vi "Client LabVIEW.vi"() -> ()   [LabVIEW 2014]
panel:
  out "ERROR":string
  out "Comptador":dbl
  out "Mínim":dbl
  out "Mitjana":dbl
  out "Waveform Chart":T1(graph)
  out "Màxim":dbl
  in  "Enviar missatge":bool
  in  "Marxa/parada":bool
  in  "Nº mostres":i32
  in  "Temps":i32 format="%02d"
  in  "Escull una acció":T2(ring)
  out "Missatge del servidor":string
  # "Marxa"
  # "Parada"
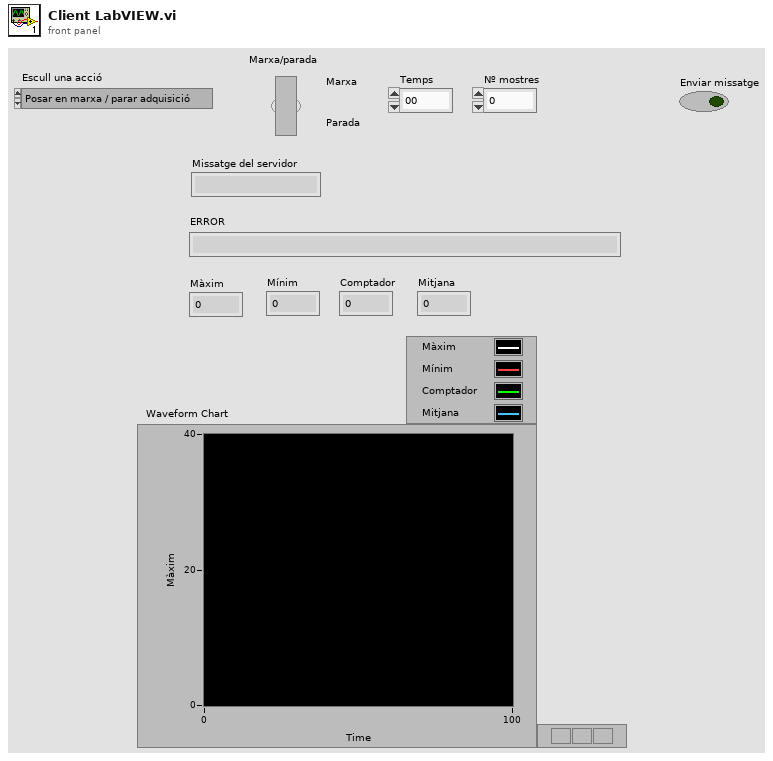
[diagram p1: front panel]
types:
  T1 = cluster{"Màxim":dbl, "Mínim":dbl, "Comptador":dbl, "Mitjana":dbl}
  T2 = enum16{"Posar en marxa / parar adquisició", "Demanar la mitjana", "Demanar màxim", "Demanar mínim", "Reset màxim/mínim", " Nombre de mostres guardades"}
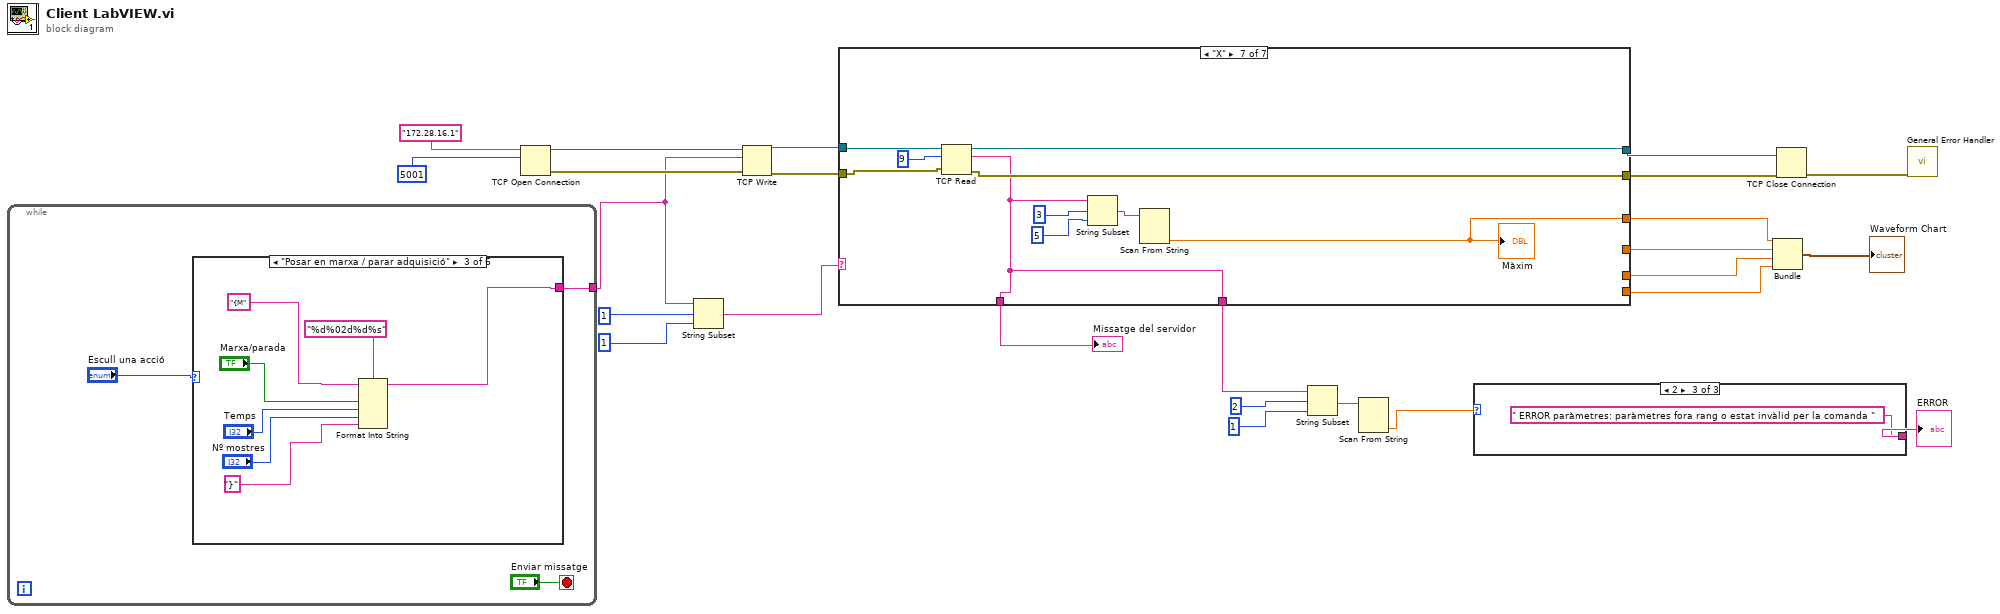
[diagram p0: block diagram]
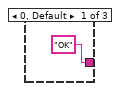
[diagram p2: hidden frame]
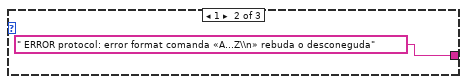
[diagram p3: hidden frame]
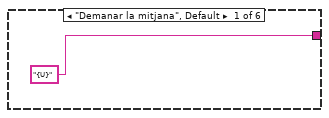
[diagram p4: hidden frame]
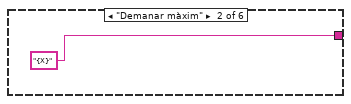
[diagram p5: hidden frame]
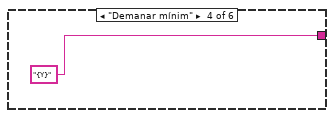
[diagram p6: hidden frame]
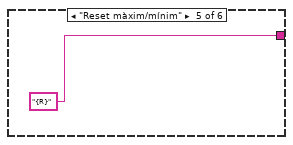
[diagram p7: hidden frame]
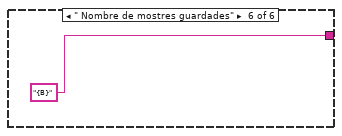
[diagram p8: hidden frame]
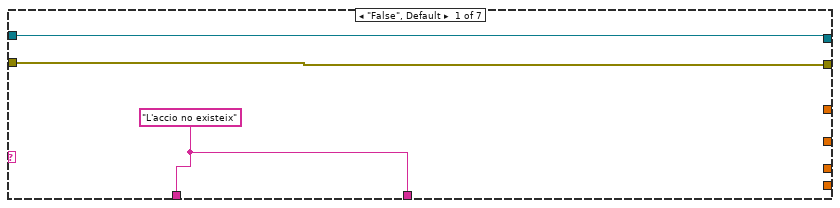
[diagram p9: hidden frame]
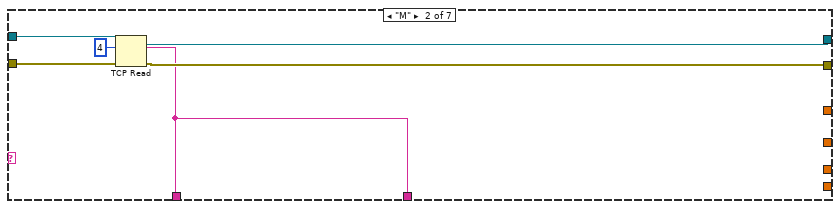
[diagram p10: hidden frame]
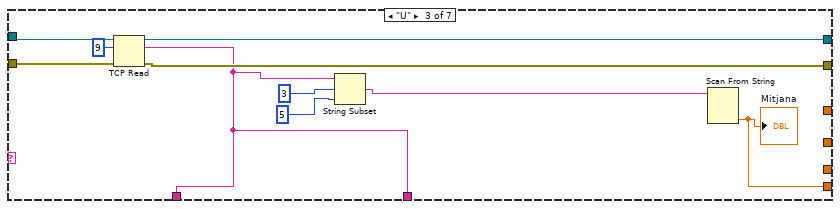
[diagram p11: hidden frame]
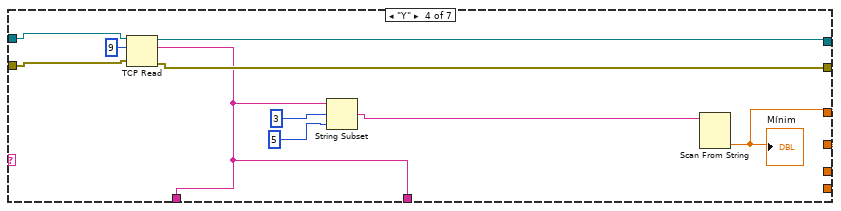
[diagram p12: hidden frame]
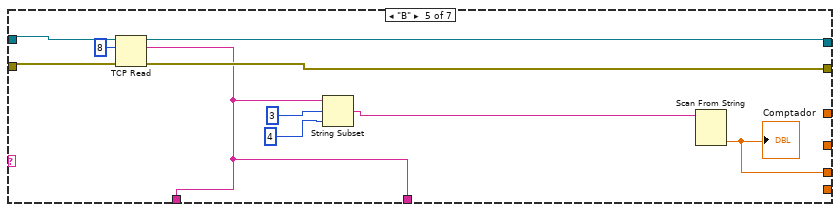
[diagram p13: hidden frame]
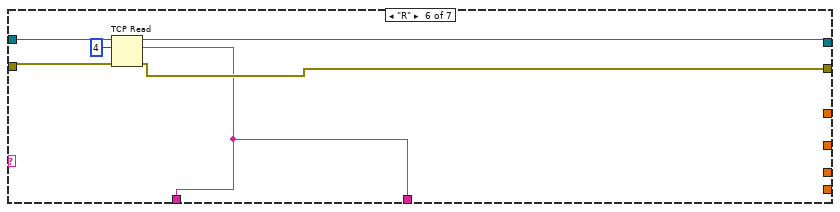
[diagram p14: hidden frame]
diagram:
  n1 = while {
    tunnel: [w27] -> w13
    stop <- "Enviar missatge" stop-if-true
    n2 = case shown="\"Posar en marxa / parar adquisició\"" "Escull una acció" {
      tunnel: ["{U}" "{X}" w31 "{Y}" "{R}" "{B}"] -> w27
      frame "Demanar la mitjana", Default {
      }
      frame "Demanar màxim" {
      }
      frame "Posar en marxa / parar adquisició" {
        n3 = Format Into String(format string="%d%02d%d%s", initial string="{M", "Marxa/parada", "Temps", "Nº mostres", "}") -> (resulting string=w31:string)  [unwired: 1 in, 1 out]
      }
      frame "Demanar mínim" {
      }
      frame "Reset màxim/mínim" {
      }
      frame " Nombre de mostres guardades" {
      }
    }
  }
  n4 = TCP Open Connection(address="172.28.16.1", remote port or service name=u16 5001) -> (connection ID=w23:refnum<k5>, error out=w22:errorcluster)  [unwired: 3 in]
  n5 = String Subset(string=w13, offset (0)=1, length (rest)=1 ("length (rest)")) -> (substring=w19:string)
  n6 = TCP Write(connection ID=w23, data in=w13, error in (no error)=w22) -> (connection ID out=w18:refnum<k5>, error out=w17:errorcluster)  [unwired: 1 in, 1 out]
  n7 = case shown="\"X\"" w19 {
    tunnel: w18 -> [w43 w48 w58 w68 w78 w84 w94]
    tunnel: w17 -> [w42 w47 w57 w67 w77 w83 w93]
    tunnel: [w43 w46 w55 w66 w76 w82 w92] -> w16
    tunnel: [w42 w45 w56 w65 w75 w81 w91] -> w15
    tunnel: [w41 w44 w51 w61 w71 w80 w87] -> w12
    tunnel: [w41 w44 w51 w61 w71 w80 w87] -> w8
    tunnel: [_ _ _ _ _ _ w86] -> w5
    tunnel: [_ _ _ w60 _ _ _] -> w4
    tunnel: [_ _ _ _ w70 _ _] -> w3
    tunnel: [_ _ w50 _ _ _ _] -> w2
    frame "False", Default {
      w41 = "L'accio no existeix" ("data out")
    }
    frame "M" {
      n8 = TCP Read(connection ID=w48, bytes to read=4, error in (no error)=w47) -> (connection ID out=w46:refnum<k5>, data out=w44:string, error out=w45:errorcluster)  [unwired: 2 in]
    }
    frame "U" {
      n9 = TCP Read(connection ID=w58, bytes to read=9, error in (no error)=w57) -> (connection ID out=w55:refnum<k5>, data out=w51:string, error out=w56:errorcluster)  [unwired: 2 in]
      n10 = String Subset(string=w51, offset (0)=3, length (rest)=5 ("offset (0)")) -> (substring=w52:string)
      n11 = Scan From String(input string=w52) -> (output 1=w50:dbl)  [unwired: 4 in, 3 out]
      "Mitjana" <- w50
    }
    frame "Y" {
      n12 = TCP Read(connection ID=w68, bytes to read=9, error in (no error)=w67) -> (connection ID out=w66:refnum<k5>, data out=w61:string, error out=w65:errorcluster)  [unwired: 2 in]
      n13 = String Subset(string=w61, offset (0)=3, length (rest)=5 ("offset (0)")) -> (substring=w62:string)
      n14 = Scan From String(input string=w62) -> (output 1=w60:dbl)  [unwired: 4 in, 3 out]
      "Mínim" <- w60
    }
    frame "B" {
      n15 = TCP Read(connection ID=w78, bytes to read=8, error in (no error)=w77) -> (connection ID out=w76:refnum<k5>, data out=w71:string, error out=w75:errorcluster)  [unwired: 2 in]
      n16 = String Subset(string=w71, offset (0)=3, length (rest)=4 ("offset (0)")) -> (substring=w72:string)
      n17 = Scan From String(input string=w72) -> (output 1=w70:dbl)  [unwired: 4 in, 3 out]
      "Comptador" <- w70
    }
    frame "R" {
      n18 = TCP Read(connection ID=w84, bytes to read=4, error in (no error)=w83) -> (connection ID out=w82:refnum<k5>, data out=w80:string, error out=w81:errorcluster)  [unwired: 2 in]
    }
    frame "X" {
      n19 = TCP Read(connection ID=w94, bytes to read=9, error in (no error)=w93) -> (connection ID out=w92:refnum<k5>, data out=w87:string, error out=w91:errorcluster)  [unwired: 2 in]
      n20 = String Subset(string=w87, offset (0)=3, length (rest)=5 ("offset (0)")) -> (substring=w88:string)
      n21 = Scan From String(input string=w88) -> (output 1=w86:dbl)  [unwired: 4 in, 3 out]
      "Màxim" <- w86
    }
  }
  "Missatge del servidor" <- w12
  n22 = String Subset(string=w8, offset (0)=2, length (rest)=1 ("offset (0)")) -> (substring=w9:string)
  n23 = Scan From String(input string=w9) -> (output 1=w1:dbl)  [unwired: 4 in, 3 out]
  n24 = case shown="2" w1 {
    tunnel: ["OK" ("ERROR") " ERROR protocol: error format comanda «A...Z\\n» rebuda o desconeguda" ("ERROR") " ERROR paràmetres: paràmetres fora rang o estat invàlid per la comanda " ("ERROR")] -> w7
    frame 0, Default {
    }
    frame 1 {
    }
    frame 2 {
    }
  }
  "ERROR" <- w7
  n25 = Bundle("Màxim"=w5, "Mínim"=w4, "Comptador"=w3, "Mitjana"=w2) -> (→"Waveform Chart":T1)  [unwired: 1 in]
  n26 = TCP Close Connection(connection ID=w16, error in (no error)=w15) -> (error out=w25:errorcluster)  [unwired: 1 in, 1 out]
  n27 = call <vilib>:"General Error Handler.vi"("error in (no error)"=w25) -> ()  [unwired: 10 in, 5 out]
